vi "measure_j-t_keithley-2450.vi"(4 "Skip pixel?":bool, 5 "Date array":string[](array[string]), 6 "Scan settings":T1={"J-V scan"=TRUE, "Start voltage (V)"=0.0, "End voltage (V)"=0.0, "Step voltage (V)"=1.4, "Scan both directions"=TRUE, "Inverted device structure"=FALSE, "Measurement delay (ms)"=10.0, "Measurement speed"=0, "Scan rate (V/s)"=0.0, "Stabilisation time (s)"=0.0, "Stabilisation mode"=0, "Stabilisation value (V or A) "=1.0, "Illumination"=0, "Stabilisation in the dark?"=FALSE, "Repeat light scans"=FALSE, "No. of repeat scans"=0.0, "Only repeat for best pixel"=1, "J-t scan"=FALSE, "J-t best pixel only"=7, "J-t start voltage (V)"=0.0, "J-t end voltage (V)"=1.4, "J-t step voltage (V)"=0.01, "Step time (s)"=0.7, "J-t scan both directions"=TRUE, "J-t inverted device structure"=FALSE, "J-t settling delay (s)"=0.0, "J-t measurement speed"=0, "J-t illumination"=2, "Max. power stabilisation"=FALSE, "Max power best pixel only"=1, "Max. power point tracker"=FALSE, "Vmp from J-V scan"=FALSE, "Max P stab. Specific voltage"=FALSE, "Vmp (V)"=1.0, "Stabilisation time step (s)"=1.0, "Total stabilisation time (s)"=100.0} {"J-t settling delay (s)" min=10.0; "J-t illumination" items=["Light only", "Dark only", "Light then dark", "Dark then light"]; "Measurement speed" items=["Fast", "Normal", "High accuracy"]; "Illumination" items=["Light only", "Dark only", "Light then dark", "Dark then light"]; "Only repeat for best pixel" items=["only for best pixel", "for best 2 pixels", "for best 3 pixels", "for best 4 pixels", "for best 5 pixels", "for best 6 pixels", "for best 7 pixels", "for all pixels"]; "No. of repeat scans" min=1.0 step=1.0; "Max power best pixel only" items=["only the best pixel", "the best 2 pixels", "the best 3 pixels", "the best 4 pixels", "the best 5 pixels", "the best 6 pixels", "the best 7 pixels", "all pixels"]; "J-t best pixel only" items=["only the best pixel", "the best 2 pixels", "the best 3 pixels", "the best 4 pixels", "the best 5 pixels", "the best 6 pixels", "the best 7 pixels", "all pixels"]; "J-t measurement speed" items=["Fast", "Normal", "High Accuracy"]; "Stabilisation mode" items=["V", "I"]; "Measurement delay (ms)" min=10.0}, 7 "Cell details cluster":T2={"Cell Position"=16, "Cell Label"="", "Pixel to measure"=0, "Area (cm^2)"=0.126, "Variable"="", "Variable value"="", "Scan settings in queue"=0, "Light or dark"="", "Measurement Type"=""} {"Pixel to measure" items=["All", "1", "2", "3", "4", "5", "6", "7", "8"]}, 8 "VISA resource name":refnum<visa-resource-name>="GPIB1::24::INSTR", 9 "Intensity (no. of suns)":string, 10 "Experiment Title":string, 11 "User Name":string) -> (3 "Jt Curve":cluster{"Y":dbl[], "Y":dbl[]}[](graph) caption="JV Curve")   [LabVIEW 2016]
uses:
  <instrlib>/Keithley 2450/Keithley 2450.lvlib
  TypeDefs/scan_settings.ctl
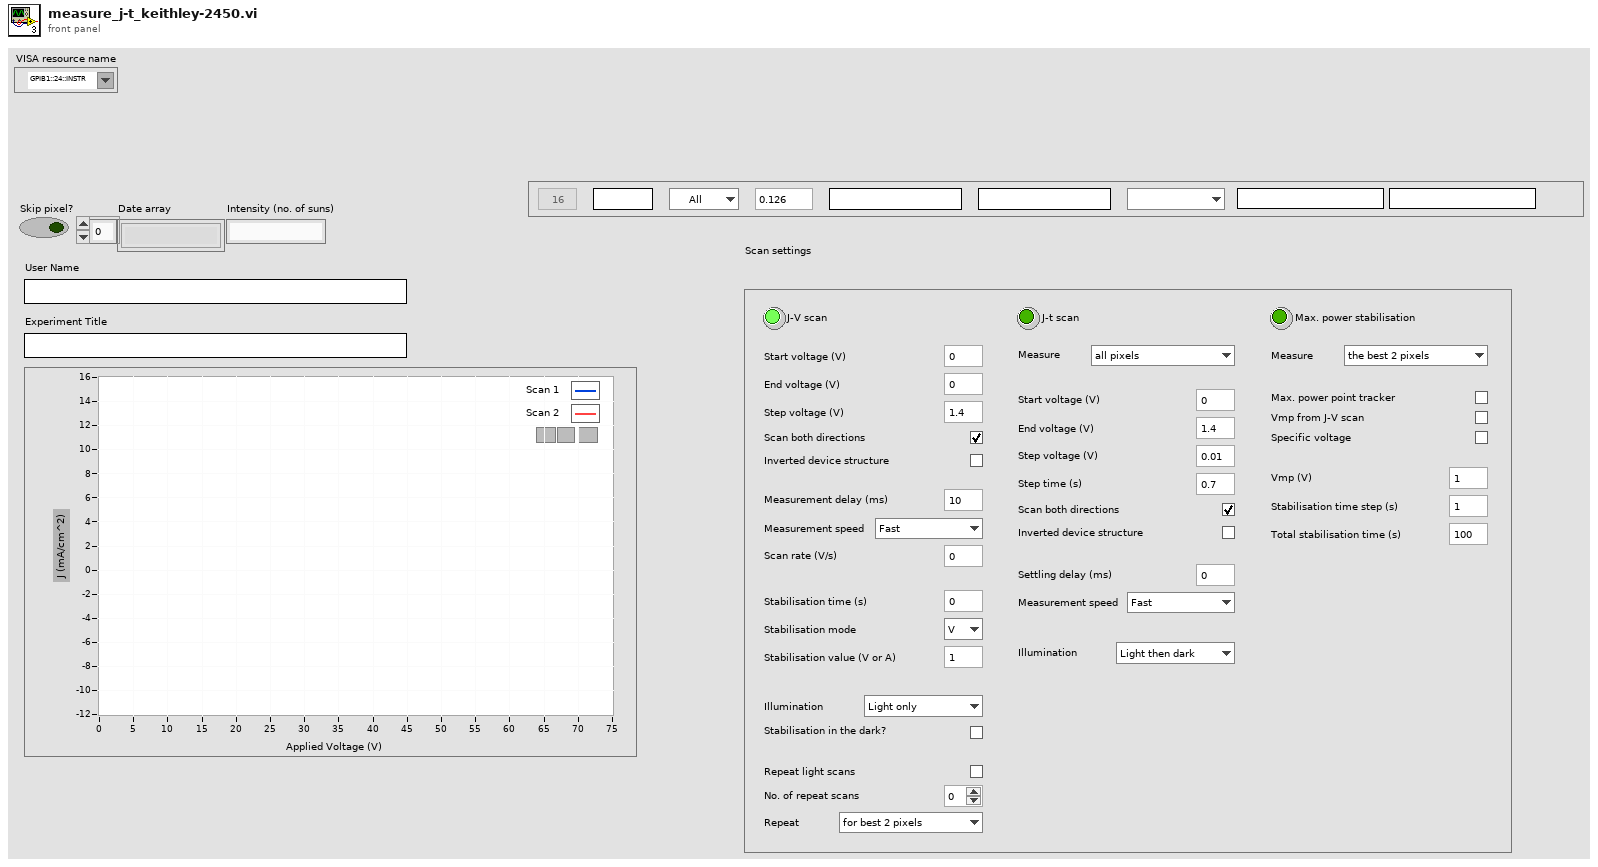
[diagram p1: front panel]
types:
  T1 = typedef "scan_settings.ctl" = cluster{"J-V scan":bool, "Start voltage (V)":dbl, "End voltage (V)":dbl, "Step voltage (V)":dbl, "Scan both directions":bool, "Inverted device structure":bool, "Measurement delay (ms)":dbl, "Measurement speed":u8, "Scan rate (V/s)":dbl, "Stabilisation time (s)":dbl, "Stabilisation mode":u16, "Stabilisation value (V or A) ":dbl, "Illumination":u16, "Stabilisation in the dark?":bool, "Repeat light scans":bool, "No. of repeat scans":dbl, "Only repeat for best pixel":u16, "J-t scan":bool, "J-t best pixel only":u16, "J-t start voltage (V)":dbl, "J-t end voltage (V)":dbl, "J-t step voltage (V)":dbl, "Step time (s)":dbl, "J-t scan both directions":bool, "J-t inverted device structure":bool, "J-t settling delay (s)":dbl, "J-t measurement speed":u16, "J-t illumination":u16, "Max. power stabilisation":bool, "Max power best pixel only":u16, "Max. power point tracker":bool, "Vmp from J-V scan":bool, "Max P stab. Specific voltage":bool, "Vmp (V)":dbl, "Stabilisation time step (s)":dbl, "Total stabilisation time (s)":dbl}
  T2 = cluster{"Cell Position":i32, "Cell Label":string, "Pixel to measure":u16, "Area (cm^2)":dbl, "Variable":string, "Variable value":string, "Scan settings in queue":u16, "Light or dark":string, "Measurement Type":string}
  T3 = typedef "imagedata.ctl" = cluster{"image type":i32, "image depth":i32, "image":u8[], "mask":u8[], "colors":u32[], "Rectangle":cluster{"left":i16, "top":i16, "right":i16, "bottom":i16}}
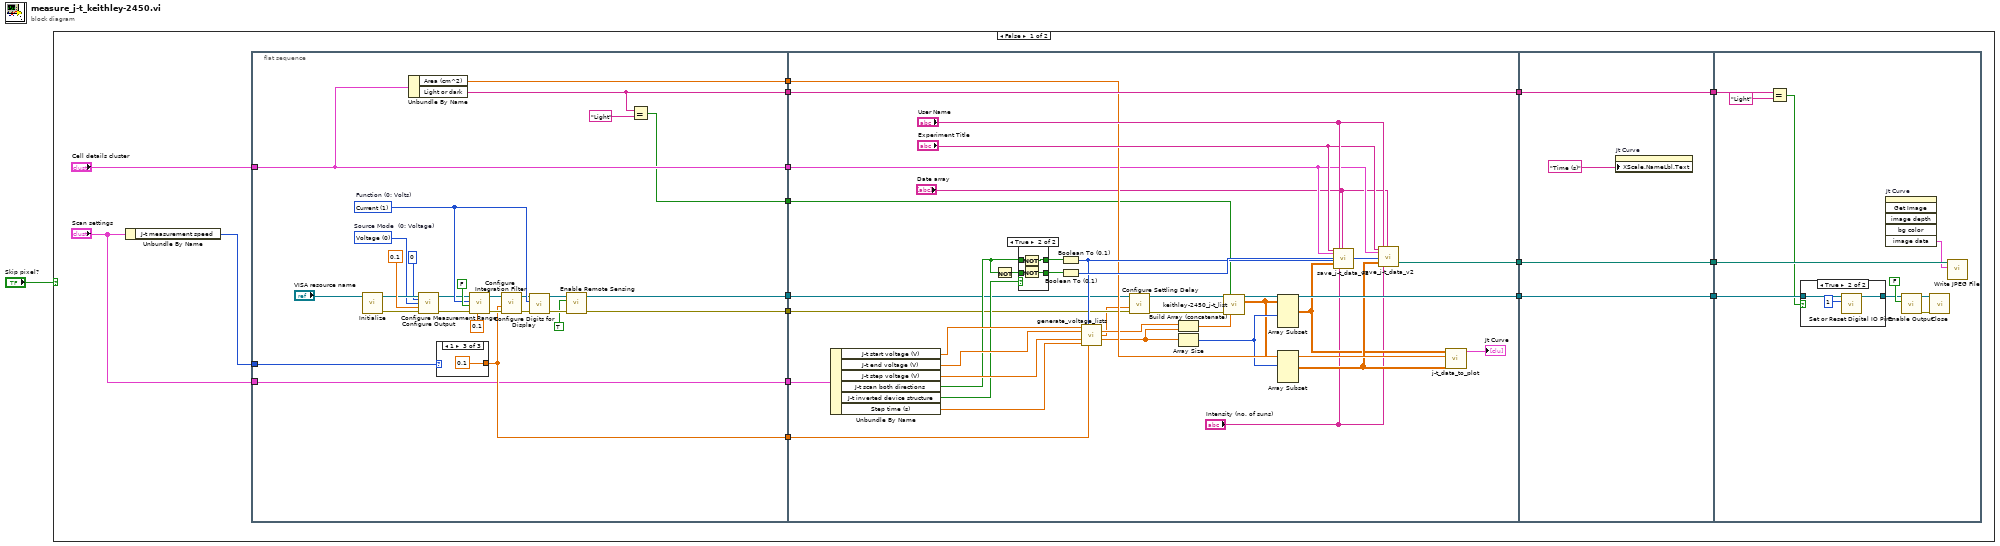
[diagram p0: block diagram]
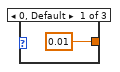
[diagram p2: hidden frame]
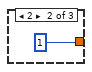
[diagram p3: hidden frame]
diagram:
  n1 = case shown="False" "Skip pixel?" {
    frame False {
      n2 = Unbundle By Name("Scan settings") -> ("J-t measurement speed"=w10:u16)
      n3 = flat-sequence {
        tunnel: [w19] -> w17
        tunnel: [w20] -> w18
        tunnel: [w38] -> w16
        tunnel: w10 -> [w37]
        tunnel: [w34] -> w15
        tunnel: "Cell details cluster" -> [w34]
        tunnel: [w36] -> w14
        tunnel: "Scan settings" -> [w36]
        tunnel: [w33] -> w13
        tunnel: [w32] -> w12
        tunnel: [w23] -> w11
        tunnel: [w62] -> w7
        tunnel: [w82] -> w5
        tunnel: w18 -> [w65]
        tunnel: w17 -> [w64]
        tunnel: w16 -> [w79]
        tunnel: w15 -> [w66]
        tunnel: w14 -> [w76]
        tunnel: [w68] -> w3
        tunnel: w13 -> [w68]
        tunnel: w12 -> [w67]
        tunnel: w11 -> [w53]
        tunnel: w7 -> [w95]
        tunnel: [w95] -> w6
        tunnel: w5 -> [w94]
        tunnel: [w94] -> w4
        tunnel: w3 -> [w93]
        tunnel: [w93] -> w2
        tunnel: w6 -> [w99]
        tunnel: w4 -> [w102]
        tunnel: w2 -> [w96]
        frame #0 {
          w21 = u16 0 items=["Voltage", "Current"]  # Source Mode  (0: Voltage)
          w39 = u16 1 items=["Volts", "Current", "Resistance"]  # Function (0: Volts)
          n4 = call <instrlib>:"Initialize.vi"("VISA resource name"="VISA resource name") -> ("error out"=w26:errorcluster, "VISA resource name out"=w27:refnum<visa-resource-name>)  [unwired: 9 in]
          n5 = Unbundle By Name(w34) -> ("Area (cm^2)"=w32:dbl, "Light or dark"=w33:string)
          n6 = call <instrlib>:"Configure Output.vi"("VISA resource name"=w27, "Source Level (0)"=0, "Source Mode  (0: Voltage)"=w21, "Source Limit Level (0.1)"=0.1, "error in (no error)"=w26) -> ("VISA resource name out"=w25:refnum<visa-resource-name>, "error out"=w24:errorcluster)  [unwired: 9 in]
          n7 = case shown="1" w37 {
            tunnel: [0.01 1 0.1] -> w38
            frame 0, Default {
            }
            frame 2 {
            }
            frame 1 {
            }
          }
          n8 = call <instrlib>:"Configure Measurement Range.vi"("Manual Range (1.0)"=0.1, "error in (no error)"=w24, "Enable Auto Range (T:Enable)"=FALSE, "Function (0: Volts)"=w39, "VISA resource name"=w25) -> ("error out"=w42:errorcluster, "VISA resource name out"=w41:refnum<visa-resource-name>)  [unwired: 5 in]
          n9 = call <instrlib>:"Configure Integration Filter.vi"("error in (no error)"=w42, "Measurement Speed (1 PLC)"=w38, "VISA resource name"=w41) -> ("error out"=w30:errorcluster, "VISA resource name out"=w31:refnum<visa-resource-name>)  [unwired: 7 in]
          n10 = call <instrlib>:"Configure Digits for Display.vi"("error in (no error)"=w30, "Function (0: Volts)"=w39, "VISA resource name"=w31) -> ("error out"=w44:errorcluster, "VISA resource name out"=w43:refnum<visa-resource-name>)  [unwired: 7 in]
          n11 = call <instrlib>:"Enable Remote Sensing.vi"("error in (no error)"=w44, "Enable Remote Sensing (T: Enable)"=TRUE ("Enable Output (T: Enable)"), "VISA resource name"=w43) -> ("error out"=w19:errorcluster, "VISA resource name out"=w20:refnum<visa-resource-name>)  [unwired: 7 in]
          n12 = Equal?(x=w33, y="Light") -> (x = y?=w23:bool)
        }
        frame #1 {
          n13 = Unbundle By Name(w76) -> ("J-t start voltage (V)"=w75:dbl, "J-t end voltage (V)"=w74:dbl, "J-t step voltage (V)"=w73:dbl, "J-t scan both directions"=w71:bool, "J-t inverted device structure"=w70:bool, "Step time (s)"=w72:dbl)
          n14 = Not(x=w71) -> (.not. x?=w83:bool)
          n15 = case shown="True" w70 {
            tunnel: [w87 w91] -> w85
            tunnel: [w86 w90] -> w84
            tunnel: w83 -> [w86 w89]
            tunnel: w71 -> [w87 w88]
            frame False {
            }
            frame True {
              n16 = Not(x=w88) -> (.not. x?=w91:bool)
              n17 = Not(x=w89) -> (.not. x?=w90:bool)
            }
          }
          n18 = Boolean To (0,1)(Boolean=w85) -> (0, 1=w80:i16)
          n19 = Boolean To (0,1)(Boolean=w84) -> (0, 1=w81:i16)
          n20 = call "generate_voltage_lists.vi"("MinVoltage"=w75, "Initial sweep direction"=w80, "Max Voltage"=w74, "V step"=w73, "t step"=w72, "NPLC"=w79) -> ("Voltage Forward List"=w63:dbl[], "Settling delay (s)"=w50:dbl, "Voltage Reverse List"=w61:dbl[])  [unwired: 7 in]
          n21 = call <instrlib>:"Configure Settling Delay.vi"("error in (no error)"=w64, "Manual Delay (0 sec)"=w50, "VISA resource name"=w65) -> ("error out"=w54:errorcluster, "VISA resource name out"=w56:refnum<visa-resource-name>)  [unwired: 7 in]
          n22 = Build Array (concatenate)(w63, w61) -> (w55:dbl[])
          n23 = Array Size(array=w61) -> (size(s)=w59:i32)
          n24 = call "keithley-2450_j-t_list.vi"("VISA resource name in"=w56, "Shutter open?"=w53, "error in (no error)"=w54, "Voltage List"=w55) -> ("VISA resource name out"=w62:refnum<visa-resource-name>, "Data Array"=w58:dbl[][])  [unwired: 9 in, 1 out]
          n25 = Array Subset(array=w58, length (row)=w59) -> (w57:dbl[][])  [unwired: 3 in]
          n26 = Array Subset(array=w58, index (row)=w59) -> (w60:dbl[][])  [unwired: 3 in]
          n27 = call "save_j-t_data_v2.vi"("Experiment Indicator"="Experiment Title", "Cell details cluster"=w66, 3:w80, 4:w57, "Username"="User Name", "Intensity (no. of suns)"="Intensity (no. of suns)", "Date array"="Date array") -> ()  [unwired: 11 in, 2 out]
          n28 = call "save_j-t_data_v2.vi"("Experiment Indicator"="Experiment Title", "Cell details cluster"=w66, 3:w81, 4:w60, "Username"="User Name", "Intensity (no. of suns)"="Intensity (no. of suns)", "Date array"="Date array") -> ("File path for JV image"=w82:path)  [unwired: 11 in, 1 out]
          n29 = call "j-t_data_to_plot.vi"("Data Array 2"=w60, 10:w67, "Data Array"=w57) -> ("JV Curve"=→"Jt Curve":cluster{"Y":dbl[], "Y":dbl[]}[])  [unwired: 8 in]
        }
        frame #2 {
          n30 = property on="Jt Curve" class="XYGraph (strict)"("XScale.NameLbl.Text"="Time (s)" ("Y Scale.Name Label.Text")) -> ()  [unwired: 2 in, 2 out]
        }
        frame #3 {
          n31 = Equal?(x=w96, y="Light") -> (x = y?=w97:bool)
          n32 = case shown="True" w97 {
            tunnel: w99 -> [w106 w108]
            tunnel: [w106 w107] -> w98
            frame False {
            }
            frame True {
              n33 = call <instrlib>:"Set or Reset Digital IO Pins.vi"("Digital IO Line (1)"=1, "VISA resource name"=w108) -> ("VISA resource name out"=w107:refnum<visa-resource-name>)  [unwired: 8 in, 1 out]
            }
          }
          n34 = invoke on="Jt Curve" class="XYGraph (strict)" method="Get Image"() -> ("image data"=w101:T3)  [unwired: 6 in, 5 out]
          n35 = call <instrlib>:"Enable Output.vi"("Enable Output (T: Enable)"=FALSE ("Output (Off)"), "VISA resource name"=w98) -> ("error out"=w104:errorcluster, "VISA resource name out"=w105:refnum<visa-resource-name>)  [unwired: 8 in]
          n36 = call <instrlib>:"Close.vi"("error in (no error)"=w104, "VISA resource name"=w105) -> ()  [unwired: 9 in, 1 out]
          n37 = call <vilib>:"Write JPEG File.vi"("image data"=w101, "path to JPEG file"=w102) -> ()  [unwired: 8 in, 2 out]
        }
      }
    }
    frame True {
    }
  }
